vi "Get Active Section Scalars.vi"(8 "error in":errorcluster, 11 "section ref in":T3 format="%.0x") -> (0 "error out":errorcluster, 2 "section scalars out":T1[](array[typedef]) {"Item Ref" format="%.0x"}, 3 "section ref out":T3 format="%.0x")   [LabVIEW 2018, in "FPGA Addon System Explorer.lvlib"]
uses:
  FPGA Addon System Explorer.lvlib
  <vilib>/NI Veristand/Custom Device API/Custom Device Item Ref.ctl
  Types/Output Scalar.ctl
  Addon Shared/Types/Data Type.ctl
  Addon Shared/Types/FG Action.ctl
  Addon Shared/SubVIs/Constants.vi
  <vilib>/NI/NI VeriStand Advanced SysDef API/SysDef API/SysDef.Property.Get.vi
  <vilib>/NI/NI VeriStand Advanced SysDef API/_SubVIs/SysDef.Property.Get.Variant.vi
  <vilib>/NI/NI VeriStand Advanced SysDef API/SysDef API/SysDef.Property.Set.vi
  <vilib>/NI/NI VeriStand Advanced SysDef API/_SubVIs/SysDef.Property.Set.Variant.vi
  Addon Shared/FPGA Addon Shared.lvlib
  <vilib>/NI Veristand/Custom Device API/Custom Device API.lvlib
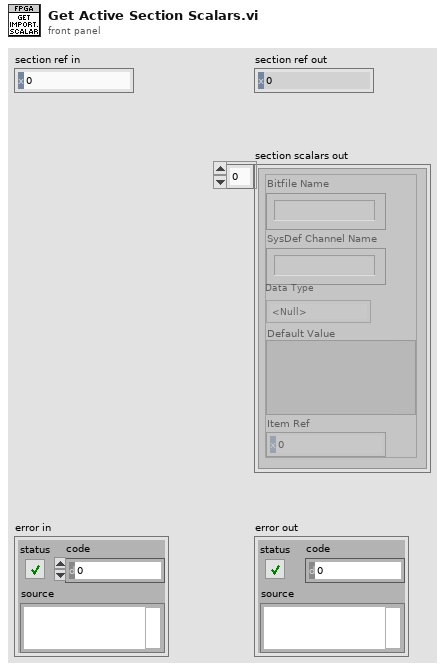
[diagram p1: front panel]
types:
  T1 = typedef "FPGA Addon System Explorer.lvlib/Output Scalar.ctl" = cluster{"Bitfile Name":string, "SysDef Channel Name":string, "Data Type":T2, "Default Value":variant, "Item Ref":T3}
  T2 = typedef "FPGA Addon Shared.lvlib/Data Type.ctl" = enum8{"<Null>", "I8", "I16", "I32", "I64", "U8", "U16", "U32", "U64", "SGL", "Boolean", "Analog PWM In Settings", "Analog PWM In", "Digital PWM In Settings", "Digital PWM In", "Digital PWM Out", "Sine Out", "FXP+/-24.5", "FXP+/-16.5", "FXP+/-32.8", "FXP+/-64.32", "FXP+/-16.7", "FXP+/-20.5", "FXP+/-27.5", "FXP+/-32.16", "FXP+16.3", "FXP+18.3", "Digital Static In", "Digital Static Out", "Digital Static In Settings", "Digital WSS Out", "Quad Encoder Settings", "Quad Encoder In", "Group"}
  T3 = typedef "Custom Device API.lvlib/Custom Device Item Ref.ctl" = u64
  T4 = typedef "FPGA Addon Shared.lvlib/FG Action.ctl" = enum8{"GET", "SET"}
  T5 = typedef "FPGA Addon Shared.lvlib/Register Information.ctl" = cluster{"Name":string, "Data Type":T2, "Default Value":variant}
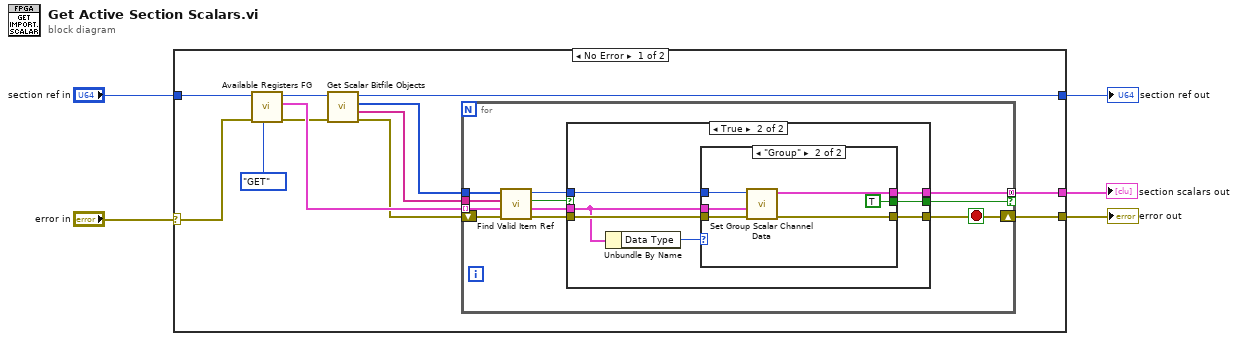
[diagram p0: block diagram]
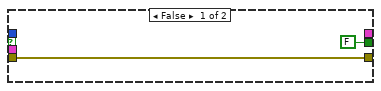
[diagram p2: hidden frame]
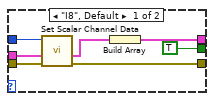
[diagram p3: hidden frame]
diagram:
  n1 = case shown="No Error" "error in" {
    selector: "error in" -> [w13 w52]
    tunnel: "section ref in" -> [w16 w51]
    tunnel: [w7 w51] -> w4
    tunnel: [w14 w52] -> w2
    tunnel: [w6 _] -> w1
    frame No Error {
      n2 = call "Available Registers FG.vi"("Action"=FG_Action."GET", "error in (no error)"=w13, "Item Ref"=w16) -> ("error out"=w11:errorcluster, "Available Registers"=w17:T5[], "Item Ref out"=w12:T3)  [unwired: 6 in]
      n3 = call "Get Scalar Bitfile Objects.vi"("error in"=w11, "item ref in"=w12) -> ("error out"=w10:errorcluster, "bitfile object names"=w9:string[], "section children refs"=w8:T3[], "item ref out"=w7:T3)  [unwired: 6 in]
      n4 = for {
        tunnel: w9 -> [w28]
        tunnel: w17 -> [w27] mode=indexing
        shift-right: [w22] -> w14
        shift-left: w10 -> [w25]
        tunnel: w8 -> [w26]
        tunnel: [w23] -> w6 mode=concatenating if=w21
        stop <- w22 stop-if-true
        n5 = call "Find Valid Item Ref.vi"("error in (no error)"=w25, "scalar channels"=w27, "bitfile object names"=w28, "section children refs"=w26) -> ("error out"=w24:errorcluster, "scalar channel out"=w19:T5, "not a ref"=w20:bool, "item ref out"=w18:T3)  [unwired: 4 in]
        n6 = case shown="True" w20 {
          tunnel: w24 -> [w30 w36]
          tunnel: [_ w35] -> w23
          tunnel: [w30 w34] -> w22
          tunnel: [FALSE w33] -> w21
          tunnel: w19 -> [_ w31]
          tunnel: w18 -> [_ w32]
          frame False {
          }
          frame True {
            n7 = Unbundle By Name(w31) -> ("Data Type"=w37:T2)
            n8 = case shown="\"Group\"" w37 {
              tunnel: w36 -> [w44 w50]
              tunnel: [w43 w49] -> w34
              tunnel: [w41 w48] -> w35
              tunnel: [TRUE TRUE] -> w33
              tunnel: w32 -> [w39 w46]
              tunnel: w31 -> [w38 w45]
              frame "I8", Default {
                n9 = call "Set Scalar Channel Data.vi"("error in (no error)"=w44, "scalar channel in"=w38, "item ref in"=w39) -> ("error out"=w43:errorcluster, "built scalar channel out"=w42:T1)  [unwired: 5 in, 2 out]
                n10 = Build Array(w42) -> (w41:T1[])
              }
              frame "Group" {
                n11 = call "Set Group Scalar Channel Data.vi"("error in (no error)"=w50, "scalar channel in"=w45, "item ref in"=w46) -> ("error out"=w49:errorcluster, "built channels out"=w48:T1[])  [unwired: 5 in]
              }
            }
          }
        }
      }
    }
    frame Error {
    }
  }
  "section ref out" <- w4
  "error out" <- w2
  "section scalars out" <- w1
